vi "To String.vi"(6 "pretty print? (F)":bool, 7 "enable LabVIEW extensions? (T)":bool=TRUE, 8 "error in (no error)":errorcluster, 11 "JSON Value in":refnum<class "JSON Value.lvclass">) -> (0 "error out":errorcluster, 3 "String":string)   [LabVIEW 2016, in "JSON Value.lvclass"]
uses:
  JSON Value.lvclass
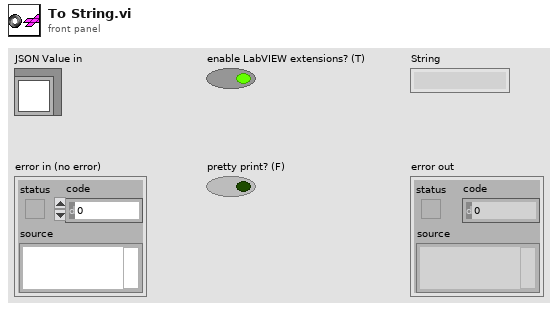
[diagram p1: front panel]
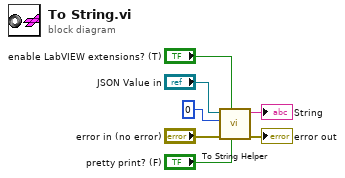
[diagram p0: block diagram]
diagram:
  n1 = call "To String Helper.vi"("pretty print? (T)"="pretty print? (F)", "enable LabVIEW extensions? (T)"="enable LabVIEW extensions? (T)", "error in (no error)"="error in (no error)", "indent"=0, "JSON Value in"="JSON Value in") -> ("error out"=→"error out":errorcluster, "String"=→"String":string)  [unwired: 5 in]
